vi "ExDebugOpenBothCamSpect.vi"() -> ()   [LabVIEW 2010]
uses:
  GlobalSpectHdl.vi
panel:
  out "Camera Open":bool
  out "Spectrometer Open":bool
  out "error out":errorcluster
  in  "error in (no error)":errorcluster
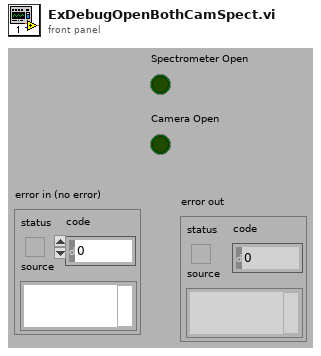
[diagram p1: front panel]
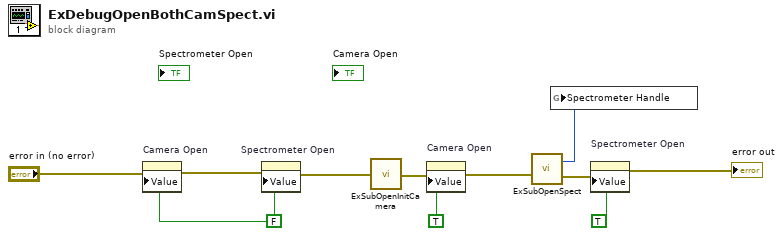
[diagram p0: block diagram]
diagram:
  w7 = FALSE
  n1 = property on="Camera Open" class="Bool (strict)"(error in="error in (no error)", "Value"=w7) -> (error out=w10:errorcluster)  [unwired: 1 in, 1 out]
  n2 = property on="Spectrometer Open" class="Bool (strict)"(error in=w10, "Value"=w7) -> (error out=w9:errorcluster)  [unwired: 1 in, 1 out]
  n3 = call "ExSubOpenInitCamera.vi"("error in (no error)"=w9) -> ("error out"=w8:errorcluster)  [unwired: 1 out]
  n4 = property on="Camera Open" class="Bool (strict)"(error in=w8, "Value"=TRUE) -> (error out=w5:errorcluster)  [unwired: 1 in, 1 out]
  n5 = call "ExSubOpenSpect.vi"("error in (no error)"=w5) -> ("Spectromete Handle"=w1:u32, "error out"=w4:errorcluster)
  n6 = global write "GlobalSpectHdl.vi" "Spectrometer Handle"(w1) -> ()
  n7 = property on="Spectrometer Open" class="Bool (strict)"(error in=w4, "Value"=TRUE) -> (error out=→"error out":errorcluster)  [unwired: 1 in, 1 out]
